vi "TurnForDegrees.vi"(8 "error in":errorcluster, 11 "Angle":dbl) -> (0 "error out":errorcluster)   [LabVIEW 2016]
uses:
  Robot Global Data.vi
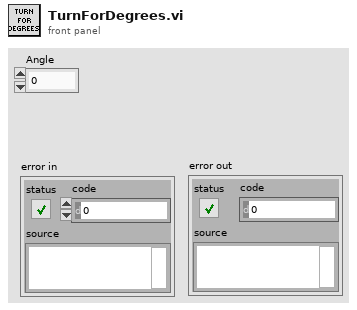
[diagram p1: front panel]
types:
  T1 = cluster{"Lower X":dbl, "Lower Y":dbl, "Upper X":dbl, "Upper Y":dbl}
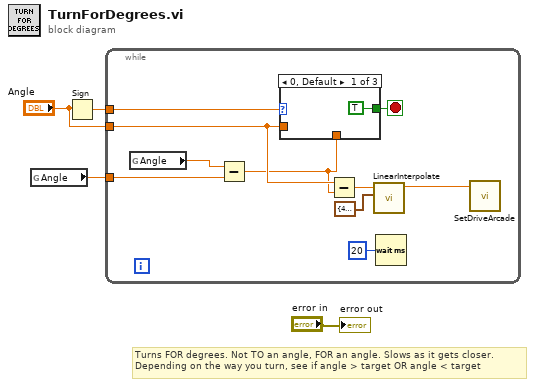
[diagram p0: block diagram]
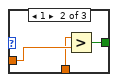
[diagram p2: hidden frame]
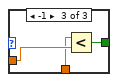
[diagram p3: hidden frame]
diagram:
  # "Turns FOR degrees. Not TO an angle, FOR an angle. Slows as it gets closer.\nDepending on the way you turn, see if angle > target OR angle < target"
  n1 = global read "Robot Global Data.vi" "Angle"() -> (w2:dbl)
  n2 = Sign(1:"Angle") -> (0:w4:dbl)
  n3 = while {
    tunnel: w4 -> [w13]
    tunnel: "Angle" -> [w9]
    tunnel: w2 -> [w11]
    stop <- w12 stop-if-true
    n4 = global read "Robot Global Data.vi" "Angle"() -> (w10:dbl)
    n5 = Subtract(x=w10, y=w11) -> (x-y=w8:dbl)
    n6 = case shown="0, Default" w13 {
      tunnel: [TRUE w18 w21] -> w12
      tunnel: w9 -> [_ w17 w20]
      tunnel: w8 -> [_ w16 w19]
      frame 0, Default {
      }
      frame 1 {
        n7 = Greater?(x=w16, y=w17) -> (0:w18:bool)
      }
      frame -1 {
        n8 = Less?(x=w19, y=w20) -> (x < y?=w21:bool)
      }
    }
    n9 = Subtract(x=w9, y=w8) -> (x-y=w7:dbl)
    n10 = call "LinearInterpolate.vi"("Config"=T1 {"Lower X"=45.0, "Lower Y"=0.55, "Upper X"=120.0, "Upper Y"=0.9}, "Value"=w7) -> ("Output"=w6:dbl)  [unwired: 9 in]
    n11 = Wait (ms)(milliseconds to wait=u32 20) -> ()  [unwired: 1 out]
    n12 = call "SetDriveArcade.vi"("Turn"=w6) -> ()  [unwired: 10 in, 1 out]
  }
  "error out" <- "error in"
